vi "recon_zern_fileIO_MATLAB.vi"(0 "Number of Phase":u32=2, 1 "Number for average":u32=2, 2 "Crop Size of image":u32=384, 3 "Background Value":u32=290, 4 "Zernike Order":u32=15, 5 "error in (no error)":errorcluster, 6 "Use GPU":bool=TRUE, 7 "Iteration Number":u32=10, 8 "File Name":string="beads_1", 9 "Gamma Value":dbl=1e-06, 10 "Path In":path=path "D:/Data", 11 "Show Input":bool, 12 "Path Out":path=path "D:/Data", 13 "Show Recon":bool=TRUE) -> (14 "Zern coef out":sgl[](array[numeric]), 16 "Time cost (s)":dbl, 17 "RMSE Value":dbl, 19 "error out":errorcluster)   [LabVIEW 2018]
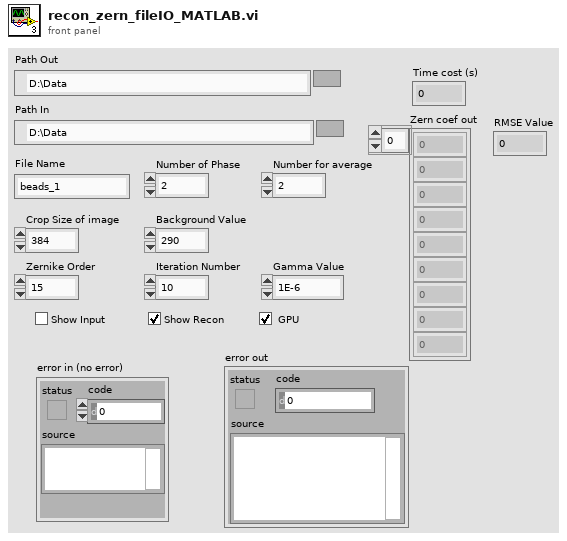
[diagram p1: front panel]
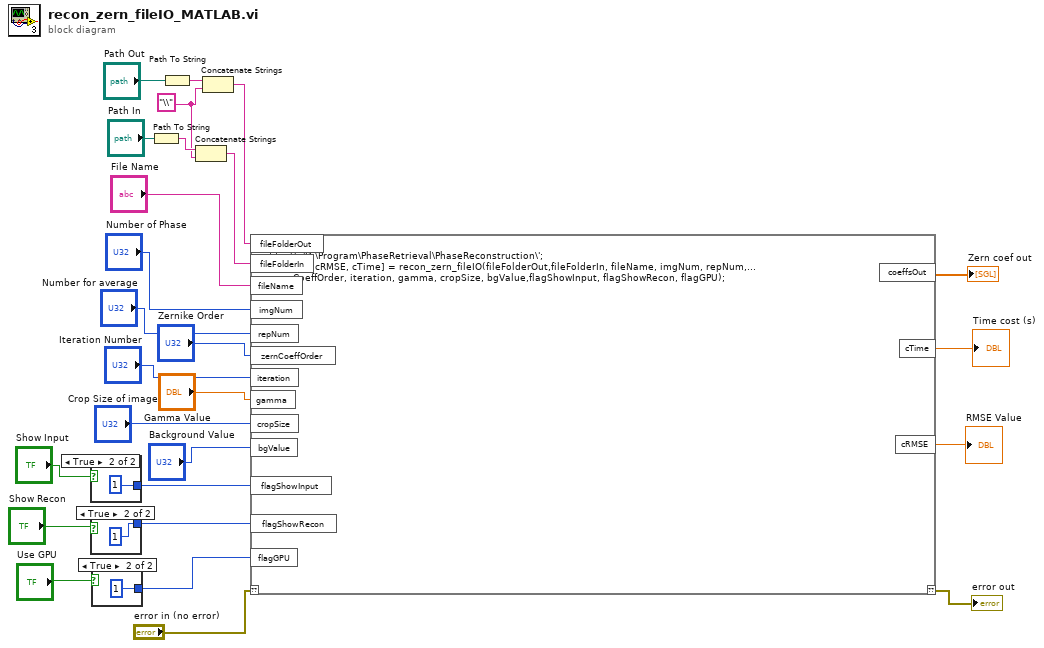
[diagram p0: block diagram]
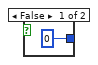
[diagram p2: hidden frame]
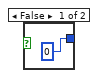
[diagram p3: hidden frame]
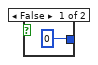
[diagram p4: hidden frame]
diagram:
  w5 = "\\"
  n1 = case shown="True" "Show Input" {
    tunnel: [0 1] -> w18
    frame False {
    }
    frame True {
    }
  }
  n2 = case shown="True" "Show Recon" {
    tunnel: [0 1] -> w17
    frame False {
    }
    frame True {
    }
  }
  n3 = case shown="True" "Use GPU" {
    tunnel: [0 1] -> w16
    frame False {
    }
    frame True {
    }
  }
  n4 = Path To String(path="Path In") -> (string=w7:string)
  n5 = Path To String(path="Path Out") -> (string=w8:string)
  n6 = Concatenate Strings(w7, w5) -> (w4:string)
  n7 = Concatenate Strings(w8, w5) -> (w6:string)
  n8 = script code="close all;\naddpath 'D:\\Program\\PhaseRetrieval\\PhaseReconstruction\\';\n[coeffsOut, cRMSE, cTime] = recon_zern_fileIO(fileFolderOut,fileFolderIn, fileName, imgNum, repNum,...\n    zernCoeffOrder, iteration, gamma, cropSize, bgValue,flagShowInput, flagShowRecon, flagGPU);"("??"="error in (no error)", "fileFolderOut"=w6, "fileFolderIn"=w4, "fileName"="File Name", "imgNum"="Number of Phase", "repNum"="Number for average", "zernCoeffOrder"="Zernike Order", "iteration"="Iteration Number", "gamma"="Gamma Value", "cropSize"="Crop Size of image", "bgValue"="Background Value", "flagShowInput"=w18, "flagShowRecon"=w17, "flagGPU"=w16) -> ("??"=→"error out":errorcluster, "coeffsOut"=→"Zern coef out":dbl[], "cTime"=→"Time cost (s)":dbl, "cRMSE"=→"RMSE Value":dbl)
